vi "BRig_dataBlock_BTPR.vi"() -> (2 "output_BTPR":i32)   [LabVIEW 2014]
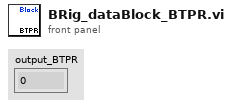
[diagram p1: front panel]
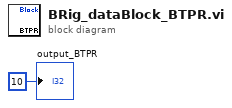
[diagram p0: block diagram]
diagram:
  "output_BTPR" <- 10 ("output_iBlock")
